vi "Configure from File.vi"(4 "digital trigger":string, 5 "acq duration (s)":dbl=0.1, 6 "clock mode":T3, 7 "acquisition mode":T4, 8 "error in (no error)":errorcluster, 9 "microphone sensitivity (dBFS)":dbl=-26.0 format="%#_13g", 10 "channels":string="PXI1Slot5\\PDMi 0", 11 "file path":path) -> (0 "error out":errorcluster, 3 "task":T1)   [LabVIEW 2022 SP3, in "Combo Digital Audio API.lvlib"]
uses:
  Combo Digital Audio API.lvlib
  <vilib>/PDM Acquisition Toolkit/host/Classes/Tasks/PDM Tasks/Controls/Acquisition Mode.ctl
  <vilib>/PDM Acquisition Toolkit/shared/controls/clock mode.ctl
  task.ctl
  controls/input type.ctl
  <vilib>/PDM Acquisition Toolkit/host/API/Controls/PDM Digital Start Trigger Cluster.ctl
  <vilib>/PDM Acquisition Toolkit/shared/controls/PXI trigger lines.ctl
  <vilib>/PDM Acquisition Toolkit/shared/controls/trigger polarity.ctl
  <vilib>/PDM Acquisition Toolkit/host/API/Public/Create Tasks/Create PCM Input Task.vi
  <vilib>/PDM Acquisition Toolkit/host/API/Public/Configure/Timing/Configure Timing - PCM Input Master.vi
  <vilib>/PDM Acquisition Toolkit/host/API/Public/Configure/PDM Channel/Configure Microphone Sensitivity DBFS - PCM Input Task.vi
  <vilib>/PDM Acquisition Toolkit/host/API/Public/Configure/Triggering/Configure PCM Input Trigger (Digital Edge).vi
  <vilib>/PDM Acquisition Toolkit/host/API/Public/Start/Start PCM Input Task.vi
  task conversion/From PCM task.vi
  <vilib>/PDM Acquisition Toolkit/host/API/Public/Create Tasks/Create PDM Input Task.vi
  <vilib>/PDM Acquisition Toolkit/host/API/Public/Configure/Timing/Configure Timing - PDM Input.vi
  <vilib>/PDM Acquisition Toolkit/host/API/Public/Configure/PDM Channel/Configure Microphone Sensitivity DBFS.vi
  <vilib>/PDM Acquisition Toolkit/host/API/Public/Configure/Triggering/Configure PDM Trigger (Digital Edge).vi
  task conversion/From PDM task.vi
  input configuration file/input cfg file.lvlib
  input configuration file/digital serial/digital serial input cfg file.lvlib
  <vilib>/PDM Acquisition Toolkit/host/API/PDM Acquisition Toolkit.lvlib
  task conversion/DAAG task conversion.lvlib
  input configuration file/PDM/PDM input cfg file.lvlib
  <vilib>/PDM Acquisition Toolkit/shared/PDM Shared.lvlib
  <vilib>/PDM Acquisition Toolkit/host/Classes/Tasks/PDM Tasks/PDM Task.lvclass
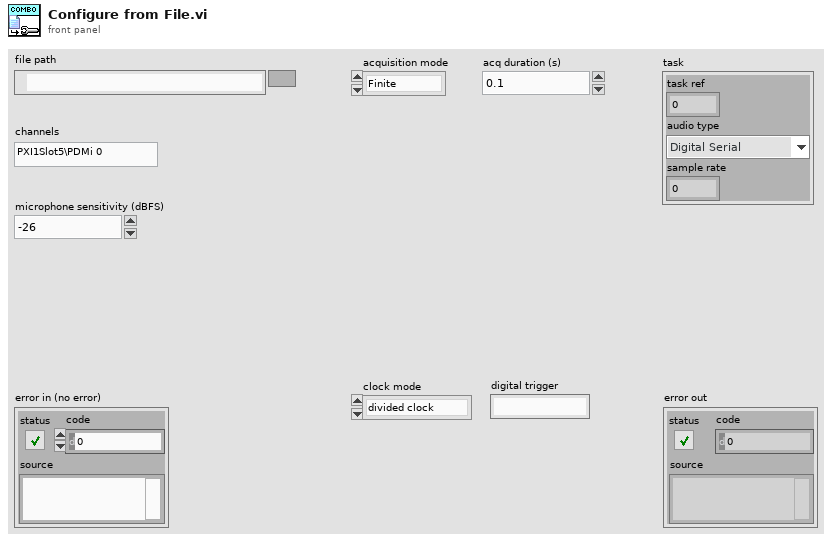
[diagram p1: front panel]
types:
  T1 = typedef "Combo Digital Audio API.lvlib/task.ctl" = cluster{"task ref":u64, "audio type":T2, "sample rate":dbl}
  T2 = typedef "input type.ctl" = enum32{"Digital Serial", "PDM"}
  T3 = typedef "PDM Shared.lvlib/clock mode.ctl" = enum16{"divided clock", "DDS"}
  T4 = typedef "PDM Acquisition Class Library.lvlib/PDM Task.lvclass/Acquisition Mode.ctl" = enum16{"Finite", "Continuous"}
  T5 = typedef "PDM Acquisition Toolkit.lvlib/PDM Digital Start Trigger Cluster.ctl" = cluster{"source":T6, "polarity":T7}
  T6 = typedef "PDM Shared.lvlib/PXI trigger lines.ctl" = enum16{"PXI_Trig0", "PXI_Trig1", "PXI_Trig2", "PXI_Trig3", "PXI_Trig4", "PXI_Trig5", "PXI_Trig6", "PXI_Trig7"}
  T7 = typedef "PDM Shared.lvlib/trigger polarity.ctl" = enum16{"Rising Edge", "Falling Edge"}
  T8 = typedef "digital serial input settings.ctl" = cluster{"number of channels":u32, "data justification":T9, "endianness":T10, "channel length":u32, "bit depth":u32, "frame clock rate":dbl, "bit clock edge sync":T11, "master clock source":T12, "master clock rate":dbl, "Logic Level":T13, "frame sync edge for channel 0":T11, "Channel 0 Offset":u32}
  T9 = typedef "PDM Shared.lvlib/PCM Data Justification.ctl" = enum16{"Left Justified", "Right Justified"}
  T10 = typedef "PDM Shared.lvlib/PCM Bit Endianness.ctl" = enum16{"MSB First", "LSB First"}
  T11 = typedef "PDM Shared.lvlib/Digital Edge.ctl" = enum8{"Rising", "Falling"}
  T12 = typedef "master clock source.ctl" = enum32{"Internal", "External"}
  T13 = typedef "PDM Acquisition Class Library.lvlib/DecoderSession.lvclass/Logic Levels.ctl" = enum16{"3.3 V", "1.8 V", "1.2 V"}
  T14 = typedef "PDM Shared.lvlib/PCM Frame Sync Control.ctl" = cluster{"Frame Length":u16, "Frame Sync Pulse Width":u16, "Bit Clock Edge  Sync":T11}
  T15 = typedef "PDM Shared.lvlib/PCM Data Format Configuration.ctl" = cluster{"Frame Sync Edge for Channel 0":T11, "Channel Count Per Frame":u8, "Channel Length":u16, "Bit Depth":u8, "Channel 0 Offset":u16, "Endianness":T10, "Data Justification":T9}
  T16 = typedef "PDM Acquisition Class Library.lvlib/PCM Input Task.lvclass/DVR PCM Input Task.ctl" = refnum<data-value>
  T17 = typedef "PDM input settings.ctl" = cluster{"PDM clock rate":dbl, "decimation factor":T18, "bit clock direction":T19, "logic level":T13}
  T18 = typedef "PDM Shared.lvlib/decimation order.ctl" = u16
  T19 = typedef "bit clock direction.ctl" = enum32{"In", "Out"}
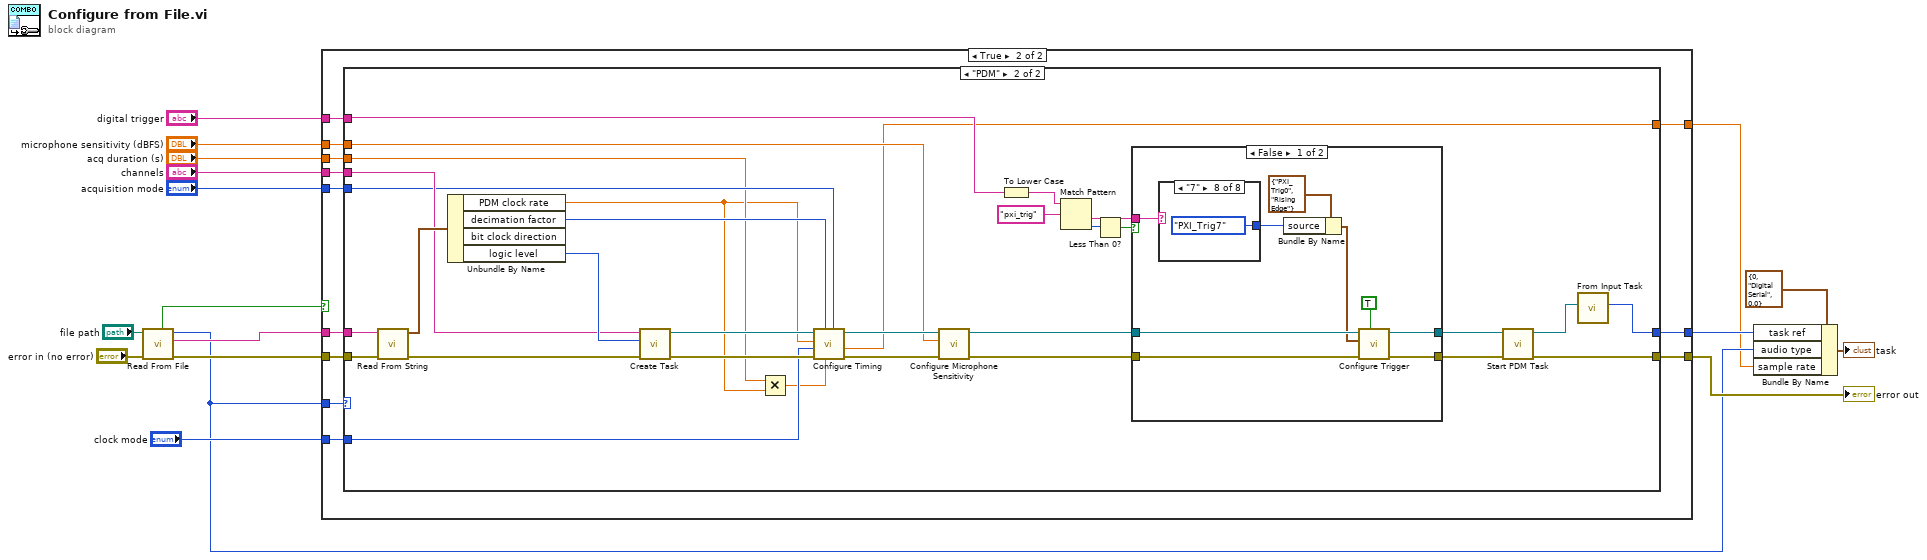
[diagram p0: block diagram]
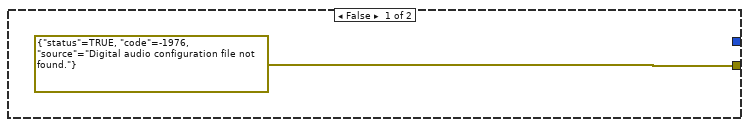
[diagram p2: hidden frame]
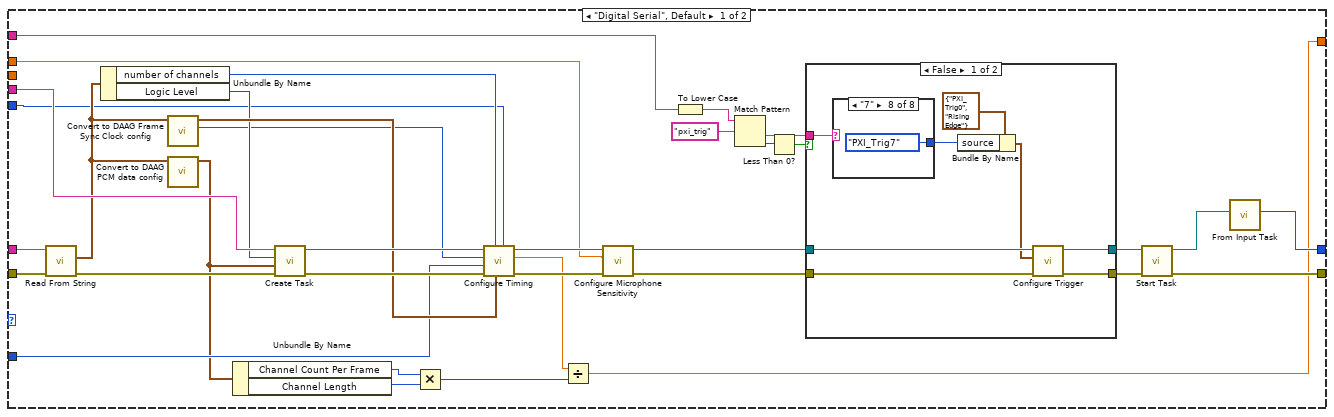
[diagram p3: hidden frame]
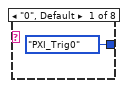
[diagram p4: hidden frame]
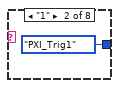
[diagram p5: hidden frame]
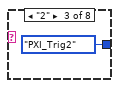
[diagram p6: hidden frame]
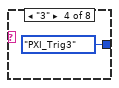
[diagram p7: hidden frame]
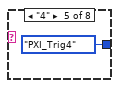
[diagram p8: hidden frame]
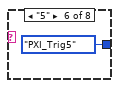
[diagram p9: hidden frame]
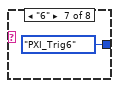
[diagram p10: hidden frame]
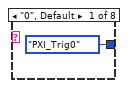
[diagram p12: hidden frame]
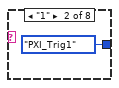
[diagram p13: hidden frame]
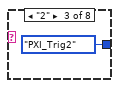
[diagram p14: hidden frame]
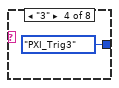
[diagram p15: hidden frame]
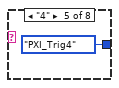
[diagram p16: hidden frame]
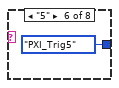
[diagram p17: hidden frame]
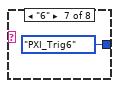
[diagram p18: hidden frame]
diagram:
  n1 = call "Read From File.vi"("error in (no error)"="error in (no error)", "file path"="file path") -> ("error out"=w17:errorcluster, "input cfg JSON"=w12:string, "input type"=w4:T2, "file exists?"=w7:bool)  [unwired: 6 in]
  n2 = case shown="True" w7 {
    tunnel: w17 -> [_ w30]
    tunnel: w4 -> [_ w29]
    tunnel: "acquisition mode" -> [_ w28]
    tunnel: "microphone sensitivity (dBFS)" -> [_ w27]
    tunnel: "acq duration (s)" -> [_ w26]
    tunnel: "channels" -> [_ w25]
    tunnel: w12 -> [_ w24]
    tunnel: "clock mode" -> [_ w23]
    tunnel: [_ w22] -> w5
    tunnel: [errorcluster {"status"=TRUE, "code"=-1976, "source"="Digital audio configuration file not found."} ("error out") w21] -> w8
    tunnel: "digital trigger" -> [_ w20]
    tunnel: [_ w19] -> w1
    frame False {
    }
    frame True {
      n3 = case shown="\"PDM\"" w29 {
        tunnel: w30 -> [w65 w114]
        tunnel: w24 -> [w64 w113]
        tunnel: w26 -> [_ w86]
        tunnel: w25 -> [w57 w106]
        tunnel: [w58 w103] -> w21
        tunnel: w27 -> [w52 w102]
        tunnel: [w49 w100] -> w22
        tunnel: w28 -> [w48 w99]
        tunnel: w23 -> [w47 w98]
        tunnel: w20 -> [w39 w88]
        tunnel: [w31 w87] -> w19
        frame "Digital Serial", Default {
          n4 = call "Read From String.vi"("error in (no error)"=w65, "JSON string"=w64) -> ("error out"=w63:errorcluster, "digital serial input settings"=w56:T8)  [unwired: 8 in]
          n5 = Unbundle By Name(w56) -> ("number of channels"=w54:u32, "Logic Level"=w53:T13)
          n6 = call "Convert to DAAG Frame Sync Clock config.vi"("digital serial input settings"=w56) -> ("Bit Clock rate"=w51:u32, "Frame Sync Clock Control"=w55:T14)  [unwired: 9 in]
          n7 = call "Convert to DAAG PCM data config.vi"("digital serial input settings"=w56) -> ("PCM data configuration"=w36:T15)  [unwired: 10 in]
          n8 = Unbundle By Name(w36) -> ("Channel Count Per Frame"=w35:u8, "Channel Length"=w34:u16)
          n9 = call-poly <vilib>:"Create Task.vi"("error in"=w63, "PCM data configuration"=w36, "logic level"=w53, "channel list"=w57) -> ("error out"=w61:errorcluster, "PCM input task out"=w62:T16)  [unwired: 6 in]
          n10 = Multiply(x=w35, y=w34) -> (x*y=w32:u16)
          n11 = call-poly <vilib>:"Configure Timing.vi"("acquisition mode"=w48, "Frame Sync Clock Control"=w55, "number of words per channel"=w54, "error in"=w61, "clock mode"=w47, "Bit Clock rate"=w51, "PCM input task in"=w62) -> ("error out"=w59:errorcluster, "actual Bit Clock rate"=w33:sgl, "PCM input task out"=w60:T16)  [unwired: 2 in]
          n12 = Divide(x=w33, y=w32) -> (x/y=w31:sgl)
          n13 = call-poly <vilib>:"Configure Microphone Sensitivity.vi"("error in"=w59, "microphone sensitivity (dBFS)"=w52, "PCM input task in"=w60) -> ("error out"=w46:errorcluster, "PCM input task out"=w45:T16)  [unwired: 7 in]
          n14 = To Lower Case(string=w39) -> (all lower case string=w38:string)
          n15 = Match Pattern(string=w38, regular expression="pxi_trig") -> (after substring=w37:string, offset past match=w41:i32)  [unwired: 1 in, 2 out]
          n16 = Less Than 0?(x=w41) -> (x < 0?=w40:bool)
          n17 = case shown="False" w40 {
            tunnel: w46 -> [w73 w82]
            tunnel: w45 -> [w72 w83]
            tunnel: [w71 w83] -> w44
            tunnel: [w70 w82] -> w43
            tunnel: w37 -> [w66 _]
            frame False {
              n18 = case shown="\"7\"" w66 {
                tunnel: [PXI_trigger_lines."PXI_Trig0" ("source") PXI_trigger_lines."PXI_Trig1" ("source") PXI_trigger_lines."PXI_Trig2" ("source") PXI_trigger_lines."PXI_Trig3" ("source") PXI_trigger_lines."PXI_Trig4" ("source") PXI_trigger_lines."PXI_Trig5" ("source") PXI_trigger_lines."PXI_Trig6" ("source") PXI_trigger_lines."PXI_Trig7" ("source")] -> w67
                frame "0", Default {
                }
                frame "1" {
                }
                frame "2" {
                }
                frame "3" {
                }
                frame "4" {
                }
                frame "5" {
                }
                frame "6" {
                }
                frame "7" {
                }
              }
              n19 = Bundle By Name(cluster=T5 {"source"=enum."PXI_Trig0", "polarity"=enum."Rising Edge"} ("trigger configuration"), "source"=w67) -> (w68:T5)
              n20 = call-poly <vilib>:"Configure Trigger.vi"("error in"=w73, "trigger configuration"=w68, "PCM input task in"=w72) -> ("error out"=w70:errorcluster, "PCM input task out"=w71:T16)  [unwired: 7 in]
            }
            frame True {
            }
          }
          n21 = call-poly <vilib>:"Start Task.vi"("error in"=w43, "PCM input task in"=w44) -> ("error out"=w58:errorcluster, "PCM input task out"=w50:T16)  [unwired: 8 in]
          n22 = call-poly "From Input Task.vi"("PCM input task"=w50) -> ("task"=w49:u64)  [unwired: 10 in]
        }
        frame "PDM" {
          n23 = call "Read From String.vi"("error in (no error)"=w114, "JSON string"=w113) -> ("error out"=w111:errorcluster, "input settings"=w112:T17)  [unwired: 8 in]
          n24 = Unbundle By Name(w112) -> ("PDM clock rate"=w85:dbl, "decimation factor"=w107:T18, "logic level"=w108:T13)  [unwired: 1 out]
          n25 = call-poly <vilib>:"Create Task.vi"("error in"=w111, "logic level"=w108, "channel list"=w106) -> ("error out"=w109:errorcluster, "PDM input task out"=w110:refnum<data-value>)  [unwired: 7 in]
          n26 = Multiply(x=w86, y=w85) -> (x*y=w84:dbl)
          n27 = call-poly <vilib>:"Configure Timing.vi"("acquisition mode"=w99, "number of PCM samples"=w84, "decimation factor"=w107, "error in"=w109, "clock mode"=w98, "PDM clock rate"=w85, "PDM input task in"=w110) -> ("error out"=w104:errorcluster, "actual PCM clock rate"=w87:dbl, "PDM input task out"=w105:refnum<data-value>)  [unwired: 1 in, 1 out]
          n28 = call-poly <vilib>:"Configure Microphone Sensitivity.vi"("error in"=w104, "microphone sensitivity (dBFS)"=w102, "PDM input task in"=w105) -> ("error out"=w92:errorcluster, "PDM input task out"=w91:refnum<data-value>)  [unwired: 7 in]
          n29 = To Lower Case(string=w88) -> (all lower case string=w94:string)
          n30 = Match Pattern(string=w94, regular expression="pxi_trig") -> (after substring=w93:string, offset past match=w96:i32)  [unwired: 1 in, 2 out]
          n31 = Less Than 0?(x=w96) -> (x < 0?=w95:bool)
          n32 = case shown="False" w95 {
            tunnel: w92 -> [w123 w132]
            tunnel: w91 -> [w122 w133]
            tunnel: [w121 w133] -> w90
            tunnel: [w120 w132] -> w89
            tunnel: w93 -> [w116 _]
            frame False {
              n33 = case shown="\"7\"" w116 {
                tunnel: [PXI_trigger_lines."PXI_Trig0" ("source") PXI_trigger_lines."PXI_Trig1" ("source") PXI_trigger_lines."PXI_Trig2" ("source") PXI_trigger_lines."PXI_Trig3" ("source") PXI_trigger_lines."PXI_Trig4" ("source") PXI_trigger_lines."PXI_Trig5" ("source") PXI_trigger_lines."PXI_Trig6" ("source") PXI_trigger_lines."PXI_Trig7" ("source")] -> w117
                frame "0", Default {
                }
                frame "1" {
                }
                frame "2" {
                }
                frame "3" {
                }
                frame "4" {
                }
                frame "5" {
                }
                frame "6" {
                }
                frame "7" {
                }
              }
              n34 = Bundle By Name(cluster=T5 {"source"=enum."PXI_Trig0", "polarity"=enum."Rising Edge"} ("trigger configuration"), "source"=w117) -> (w118:T5)
              n35 = call-poly <vilib>:"Configure Trigger.vi"("remove filter delay samples"=TRUE, "error in"=w123, "trigger configuration"=w118, "PDM input task in"=w122) -> ("error out"=w120:errorcluster, "PDM input task out"=w121:refnum<data-value>)  [unwired: 6 in]
            }
            frame True {
            }
          }
          n36 = call <vilib>:"Start PDM Task.vi"("error in"=w89, "PDM input task in"=w90) -> ("error out"=w103:errorcluster, "PDM input task out"=w101:refnum<data-value>)  [unwired: 8 in]
          n37 = call-poly "From Input Task.vi"("PDM input task"=w101) -> ("task"=w100:u64)  [unwired: 10 in]
        }
      }
    }
  }
  "error out" <- w8
  n38 = Bundle By Name(cluster=T1 {"task ref"=0, "audio type"=enum."Digital Serial", "sample rate"=0.0} ("task"), "task ref"=w5, "audio type"=w4, "sample rate"=w1) -> (→"task":T1)
